vi "Main.vi"   [LabVIEW 2020, in "AR Example.lvlib"]
uses:
  AR Example.lvlib
  UI/UI.lvclass
types:
  T1 = enum32{"Invalid", "Standard", "Closed", "Hidden", "Minimized", "Maximized"}
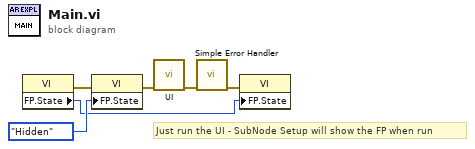
[diagram p0: block diagram]
diagram:
  # "Just run the UI - SubNode Setup will show the FP when run"
  n1 = property class="VI"() -> (error out=w2:errorcluster, "FP.State"=w1:T1)  [unwired: 2 in, 1 out]
  n2 = property class="VI"(error in=w2, "FP.State"=T1."Hidden" ("Front Panel Window:State")) -> (error out=w5:errorcluster)  [unwired: 1 in, 1 out]
  n3 = call "UI.vi"("error in"=w5) -> ("error out"=w6:errorcluster)  [unwired: 10 in]
  n4 = call <vilib>:"Simple Error Handler.vi"("error in (no error)"=w6) -> ("error out"=w4:errorcluster)  [unwired: 4 in, 4 out]
  n5 = property class="VI"(error in=w4, "FP.State"=w1) -> ()  [unwired: 1 in, 2 out]
